vi "create_model_init.vi"(8 "error in (no error)":errorcluster, 9 "ModuleModel":string[](array[string]), 10 "Icon file":path, 11 "Control Path":path) -> (0 "error out":errorcluster)   [LabVIEW 2020]
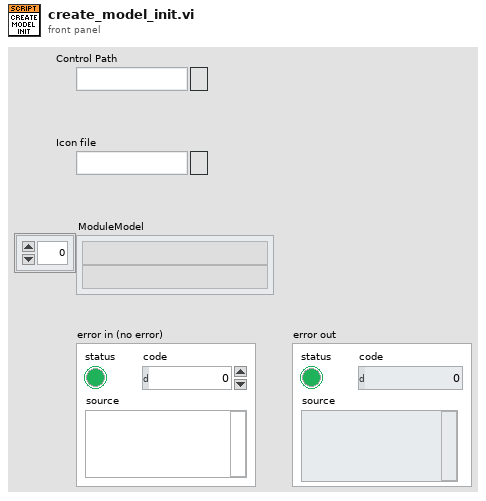
[diagram p1: front panel]
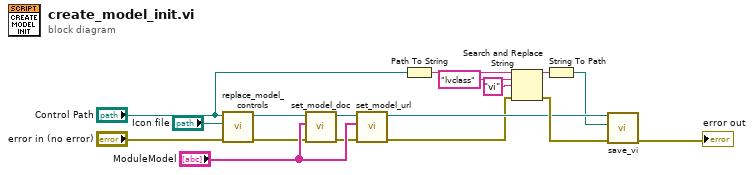
[diagram p0: block diagram]
diagram:
  n1 = call "replace_model_controls.vi"("error in (no error)"="error in (no error)", "Image File"="Icon file", "Control path"="Control Path") -> ("error out"=w3:errorcluster, "vi refnum"=w5:refnum<vi>)  [unwired: 7 in]
  n2 = call "set_model_doc.vi"("error in"=w3, "Array"="ModuleModel", "vi refnum"=w5) -> ("error out"=w4:errorcluster, "reference out"=w6:refnum<vi>)  [unwired: 7 in]
  n3 = call "set_model_url.vi"("error in (no error)"=w4, "Array in"="ModuleModel", "VI in"=w6) -> ("error out"=w10:errorcluster, "VI out"=w15:refnum<vi>)  [unwired: 7 in]
  n4 = Path To String(path="Control Path") -> (string=w9:string)
  n5 = Search and Replace String(input string=w9, search string="lvclass", replace string="vi" ("replace string (\"\")"), error in=w10) -> (result string=w14:string, error out=w16:errorcluster)  [unwired: 4 in, 2 out]
  n6 = String To Path(string=w14) -> (path=w13:path)
  n7 = call "save_vi.vi"("error in (no error)"=w16, "Path to Saved File"=w13, "VI in"=w15) -> ("error out"=→"error out":errorcluster)  [unwired: 8 in]
